vi "Write Output value.vi"(8 "error in (no error)":errorcluster, 10 "Output Value.lvclass":refnum<class "Output Value.lvclass">, 11 "Set Output Msg in":refnum<class "Set Output Msg.lvclass">) -> (0 "error out":errorcluster, 3 "Set Output Msg out":refnum<class "Set Output Msg.lvclass">)   [LabVIEW 2019, in "Set Output Msg.lvclass"]
uses:
  Set Output Msg.lvclass
  NHMFL_Core/Libraries/Utilities/Output Value/Output Value.lvclass
  Set Output Msg.lvclass/Set Output Msg.ctl
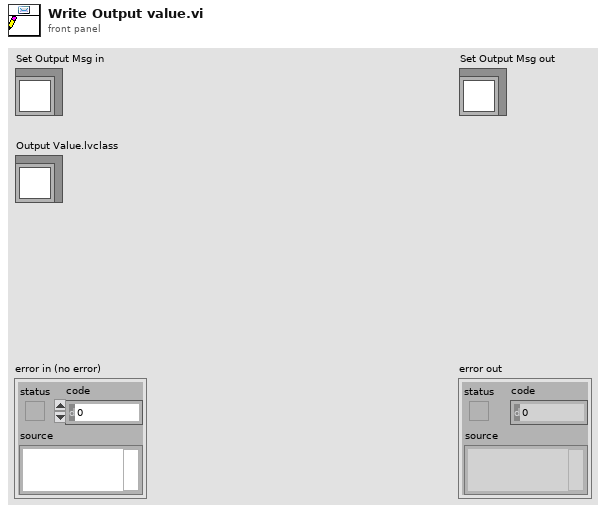
[diagram p1: front panel]
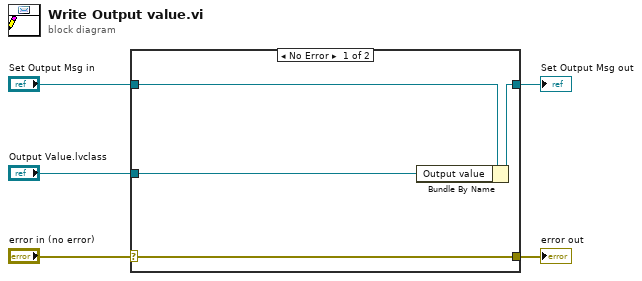
[diagram p0: block diagram]
diagram:
  n1 = case shown="No Error" "error in (no error)" {
    selector: "error in (no error)" -> [w9 w10]
    tunnel: [w9 w10] -> w4
    tunnel: [w7 w11] -> w2
    tunnel: "Set Output Msg in" -> [w8 w11]
    tunnel: "Output Value.lvclass" -> [w6 _]
    frame No Error {
      n2 = Bundle By Name(cluster=w8, "Output value"=w6) -> (w7:refnum<class "Set Output Msg.lvclass">)
    }
    frame Error {
    }
  }
  "error out" <- w4
  "Set Output Msg out" <- w2
